vi "AutoCrossSubVi.vi"(0 "AutoDriveSpeed":dbl, 1 "DistanceAutoLineToBar":dbl, 2 "BarToShootLine":dbl, 3 "DriveDistanceDeadband":dbl, 5 "DriveDistanceVDeadband":dbl, 7 "VDeadband":dbl, 9 "EncoderDevRef 2":T1, 12 "Deadband":dbl, 13 "String":string, 14 "EncoderDevRef":T1) -> ()   [LabVIEW 2015]
uses:
  <vilib>/Rock Robotics/WPI/Encoder/WPI_EncoderDevRef.ctl
  <vilib>/Rock Robotics/SystemInterfaces/Encoder/FPGA_EncoderIdx.ctl
  <vilib>/Rock Robotics/SystemInterfaces/Counter/FPGA_CounterCtrSystemIndex.ctl
  <vilib>/Rock Robotics/WPI/Encoder/WPI_EncoderType.ctl
  AutoTask/Implementation/AutoTask Setpoints.ctl
  AutoTask/Implementation/AutoTask Operations.ctl
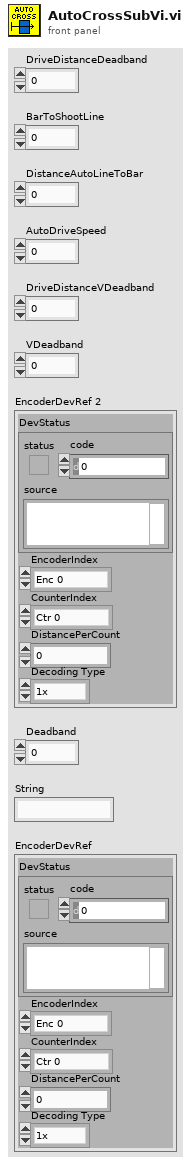
[diagram p1: front panel]
types:
  T1 = typedef "WPI_EncoderDevRef.ctl" = cluster{"DevStatus":errorcluster, "EncoderIndex":T2, "CounterIndex":T3, "DistancePerCount":dbl, "Decoding Type":T4}
  T2 = typedef "FPGA_EncoderIdx.ctl" = enum8{"Enc 0", "Enc 1", "Enc 2", "Enc 3", "Enc 4", "Enc 5", "Enc 6", "Enc 7", "Invalid"}
  T3 = typedef "FPGA_CounterCtrSystemIndex.ctl" = enum8{"Ctr 0", "Ctr 1", "Ctr 2", "Ctr 3", "Ctr 4", "Ctr 5", "Ctr 6", "Ctr 7", "Invalid"}
  T4 = typedef "WPI_EncoderType.ctl" = enum16{"1x", "2x", "4x"}
  T5 = typedef "AutoTask Setpoints.ctl" = cluster{"Operation":T6, "Setpoint":dbl, "Duration":dbl, "Speed":dbl, "Angle":dbl, "VDeadband":dbl, "Deadband":dbl}
  T6 = typedef "AutoTask Operations.ctl" = enum16{"Reserve", "Read Current", "Immediate", "DriveDistance", "AutoShoot", "FaceForward", "AutoAlign", "AutoTurn", "DriveToLine", "DriveToIncline", "DriveTillFlat"}
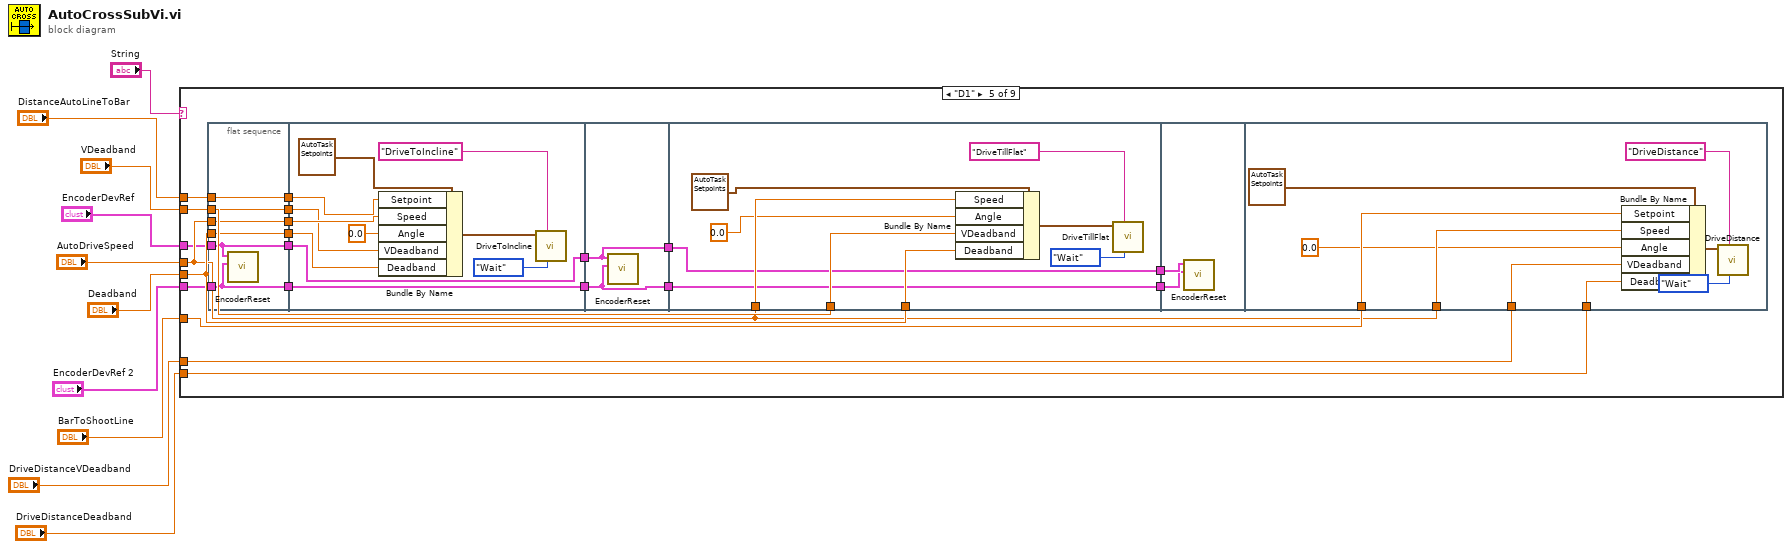
[diagram p0: block diagram]
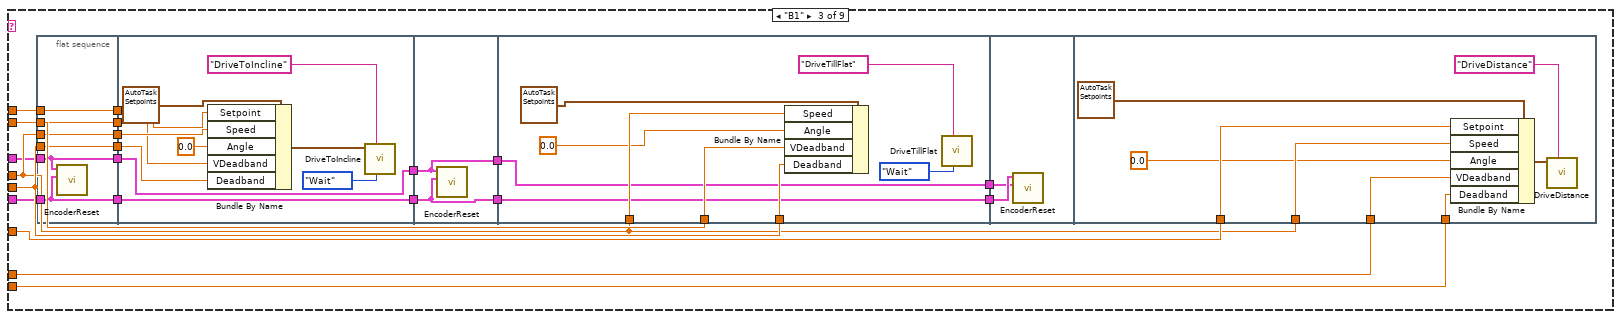
[diagram p4: hidden frame]
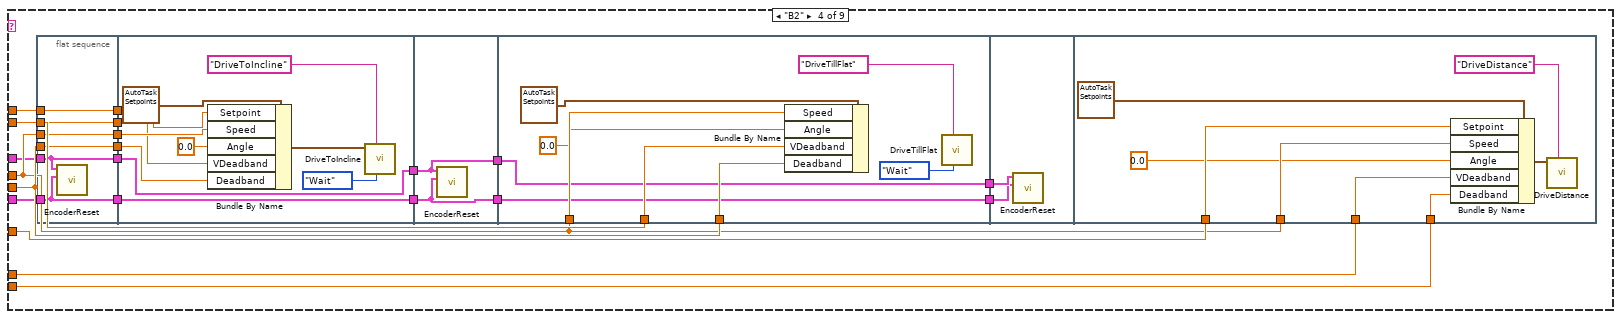
[diagram p5: hidden frame]
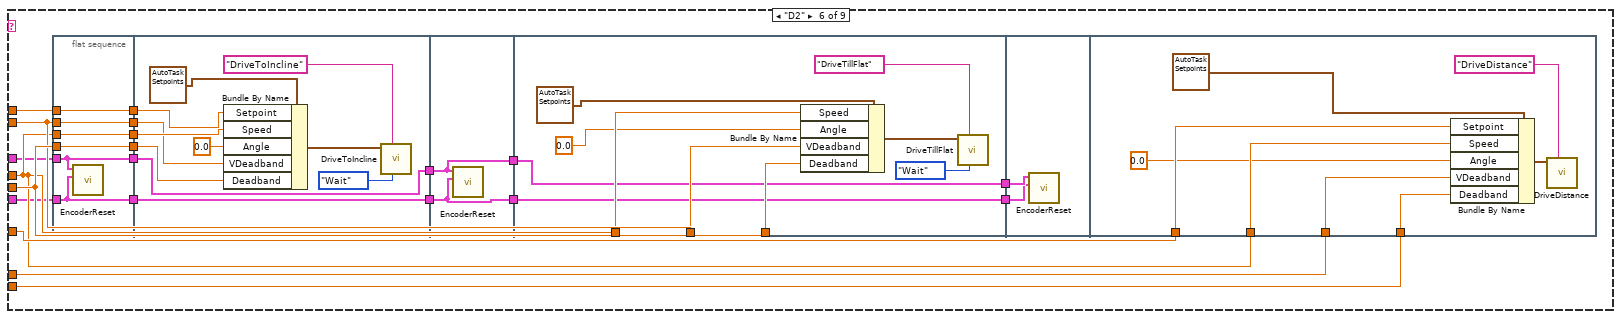
[diagram p6: hidden frame]
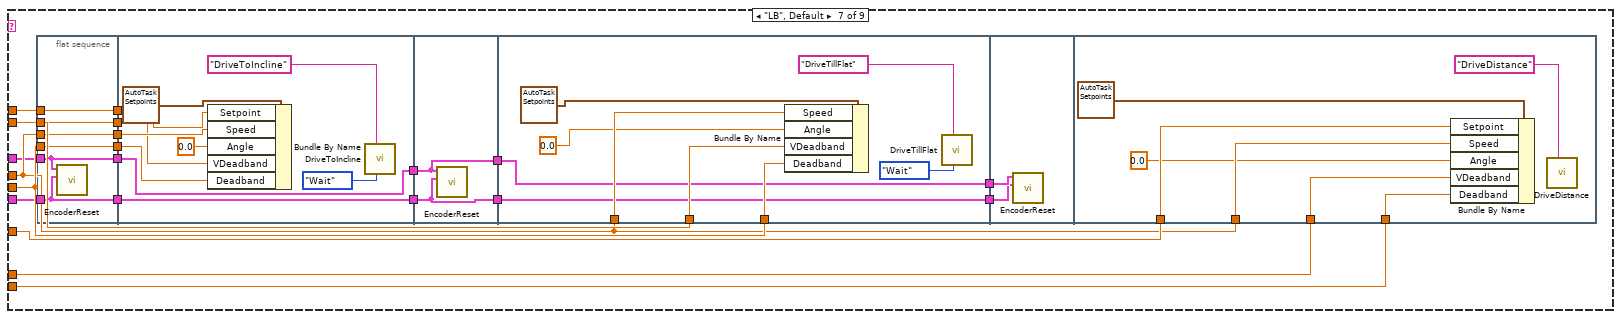
[diagram p7: hidden frame]
diagram:
  n1 = case shown="\"D1\"" "String" {
    tunnel: "DistanceAutoLineToBar" -> [_ _ w31 w90 w149 w210 w270 _ _]
    tunnel: "AutoDriveSpeed" -> [_ _ w27 w86 w145 w206 w266 _ _]
    tunnel: "VDeadband" -> [_ _ w29 w88 w147 w208 w268 _ _]
    tunnel: "Deadband" -> [_ _ w30 w89 w148 w209 w269 _ _]
    tunnel: "BarToShootLine" -> [_ _ w28 w87 w146 w207 w267 _ _]
    tunnel: "DriveDistanceDeadband" -> [_ _ w26 w85 w144 w205 w265 _ _]
    tunnel: "DriveDistanceVDeadband" -> [_ _ w25 w84 w143 w204 w264 _ _]
    tunnel: "EncoderDevRef 2" -> [_ _ w19 w78 w138 w198 w258 _ _]
    tunnel: "EncoderDevRef" -> [_ _ w20 w79 w137 w199 w259 _ _]
    frame "A1" {
    }
    frame "A2" {
    }
    frame "B1" {
      n2 = flat-sequence {
        tunnel: w30 -> [w34]
        tunnel: w29 -> [w35]
        tunnel: w27 -> [w36]
        tunnel: w31 -> [w37]
        tunnel: [w37] -> w24
        tunnel: [w36] -> w23
        tunnel: [w35] -> w22
        tunnel: [w34] -> w21
        tunnel: w20 -> [w33]
        tunnel: w19 -> [w32]
        tunnel: [w33] -> w18
        tunnel: [w32] -> w16
        tunnel: w24 -> [w45]
        tunnel: w23 -> [w44]
        tunnel: w22 -> [w42]
        tunnel: w21 -> [w41]
        tunnel: w18 -> [w39]
        tunnel: [w39] -> w17
        tunnel: w16 -> [w38]
        tunnel: [w38] -> w15
        tunnel: w17 -> [w49]
        tunnel: w15 -> [w50]
        tunnel: [w50] -> w14
        tunnel: [w49] -> w12
        tunnel: w27 -> [w56]
        tunnel: w30 -> [w54]
        tunnel: w29 -> [w53]
        tunnel: w14 -> [w52]
        tunnel: [w52] -> w13
        tunnel: w12 -> [w51]
        tunnel: [w51] -> w11
        tunnel: w13 -> [w61]
        tunnel: w11 -> [w60]
        tunnel: w28 -> [w66]
        tunnel: w27 -> [w65]
        tunnel: w26 -> [w63]
        tunnel: w25 -> [w62]
        frame #0 {
          n3 = call "EncoderReset.vi"("EncoderDevRef 2"=w32, "EncoderDevRef"=w33) -> ()  [unwired: 10 in]
        }
        frame #1 {
          n4 = Bundle By Name(cluster=T5 {"Operation"=enum."DriveToIncline", "Setpoint"=0.0, "Duration"=0.0, "Speed"=0.0, "Angle"=0.0, "VDeadband"=0.0, "Deadband"=0.0} ("SubSystem Data"), "Setpoint"=w45, "Speed"=w44, "Angle"=0.0, "VDeadband"=w42, "Deadband"=w41) -> (w47:T5)
          n5 = call "DriveToIncline.vi"("Synchronization"=enum16{"Start", "Wait"}."Wait", "Description"="DriveToIncline", "SubSystem Data"=w47) -> ()  [unwired: 8 in, 1 out]
        }
        frame #2 {
          n6 = call "EncoderReset.vi"("EncoderDevRef 2"=w50, "EncoderDevRef"=w49) -> ()  [unwired: 10 in]
        }
        frame #3 {
          n7 = Bundle By Name(cluster=T5 {"Operation"=enum."Reserve", "Setpoint"=0.0, "Duration"=0.0, "Speed"=0.0, "Angle"=0.0, "VDeadband"=0.0, "Deadband"=0.0} ("SubSystem Data"), "Speed"=w56, "Angle"=0.0, "VDeadband"=w53, "Deadband"=w54) -> ()  [unwired: 1 out]
          n8 = call "DriveTillFlat.vi"("Synchronization"=enum16{"Start", "Wait"}."Wait", "Description"="DriveTillFlat") -> ()  [unwired: 9 in, 1 out]
        }
        frame #4 {
          n9 = call "EncoderReset.vi"("EncoderDevRef 2"=w60, "EncoderDevRef"=w61) -> ()  [unwired: 10 in]
        }
        frame #5 {
          n10 = Bundle By Name(cluster=T5 {"Operation"=enum."DriveDistance", "Setpoint"=0.0, "Duration"=0.0, "Speed"=0.0, "Angle"=0.0, "VDeadband"=0.0, "Deadband"=0.0} ("SubSystem Data"), "Setpoint"=w66, "Speed"=w65, "Angle"=0.0, "VDeadband"=w62, "Deadband"=w63) -> (w68:T5)
          n11 = call "DriveDistance.vi"("Description"="DriveDistance", "SubSystem Data"=w68) -> ()  [unwired: 9 in, 1 out]
        }
      }
    }
    frame "B2" {
      n12 = flat-sequence {
        tunnel: w89 -> [w93]
        tunnel: w88 -> [w94]
        tunnel: w86 -> [w95]
        tunnel: w90 -> [w96]
        tunnel: [w96] -> w83
        tunnel: [w95] -> w82
        tunnel: [w94] -> w81
        tunnel: [w93] -> w80
        tunnel: w79 -> [w92]
        tunnel: w78 -> [w91]
        tunnel: [w92] -> w77
        tunnel: [w91] -> w75
        tunnel: w83 -> [w104]
        tunnel: w82 -> [w103]
        tunnel: w81 -> [w101]
        tunnel: w80 -> [w100]
        tunnel: w77 -> [w98]
        tunnel: [w98] -> w76
        tunnel: w75 -> [w97]
        tunnel: [w97] -> w74
        tunnel: w76 -> [w109]
        tunnel: w74 -> [w108]
        tunnel: [w109] -> w73
        tunnel: [w108] -> w71
        tunnel: w86 -> [w115]
        tunnel: w89 -> [w113]
        tunnel: w88 -> [w112]
        tunnel: w73 -> [w111]
        tunnel: [w111] -> w72
        tunnel: w71 -> [w110]
        tunnel: [w110] -> w70
        tunnel: w72 -> [w120]
        tunnel: w70 -> [w119]
        tunnel: w87 -> [w125]
        tunnel: w86 -> [w124]
        tunnel: w85 -> [w122]
        tunnel: w84 -> [w121]
        frame #0 {
          n13 = call "EncoderReset.vi"("EncoderDevRef 2"=w91, "EncoderDevRef"=w92) -> ()  [unwired: 10 in]
        }
        frame #1 {
          n14 = Bundle By Name(cluster=T5 {"Operation"=enum."DriveToIncline", "Setpoint"=0.0, "Duration"=0.0, "Speed"=0.0, "Angle"=0.0, "VDeadband"=0.0, "Deadband"=0.0} ("SubSystem Data"), "Setpoint"=w104, "Speed"=w103, "Angle"=0.0, "VDeadband"=w101, "Deadband"=w100) -> (w106:T5)
          n15 = call "DriveToIncline.vi"("Synchronization"=enum16{"Start", "Wait"}."Wait", "Description"="DriveToIncline", "SubSystem Data"=w106) -> ()  [unwired: 8 in, 1 out]
        }
        frame #2 {
          n16 = call "EncoderReset.vi"("EncoderDevRef 2"=w108, "EncoderDevRef"=w109) -> ()  [unwired: 10 in]
        }
        frame #3 {
          n17 = Bundle By Name(cluster=T5 {"Operation"=enum."Reserve", "Setpoint"=0.0, "Duration"=0.0, "Speed"=0.0, "Angle"=0.0, "VDeadband"=0.0, "Deadband"=0.0} ("SubSystem Data"), "Speed"=w115, "Angle"=0.0, "VDeadband"=w112, "Deadband"=w113) -> ()  [unwired: 1 out]
          n18 = call "DriveTillFlat.vi"("Synchronization"=enum16{"Start", "Wait"}."Wait", "Description"="DriveTillFlat") -> ()  [unwired: 9 in, 1 out]
        }
        frame #4 {
          n19 = call "EncoderReset.vi"("EncoderDevRef 2"=w119, "EncoderDevRef"=w120) -> ()  [unwired: 10 in]
        }
        frame #5 {
          n20 = Bundle By Name(cluster=T5 {"Operation"=enum."DriveDistance", "Setpoint"=0.0, "Duration"=0.0, "Speed"=0.0, "Angle"=0.0, "VDeadband"=0.0, "Deadband"=0.0} ("SubSystem Data"), "Setpoint"=w125, "Speed"=w124, "Angle"=0.0, "VDeadband"=w121, "Deadband"=w122) -> (w127:T5)
          n21 = call "DriveDistance.vi"("Description"="DriveDistance", "SubSystem Data"=w127) -> ()  [unwired: 9 in, 1 out]
        }
      }
    }
    frame "D1" {
      n22 = flat-sequence {
        tunnel: w148 -> [w152]
        tunnel: w147 -> [w153]
        tunnel: w145 -> [w154]
        tunnel: w149 -> [w155]
        tunnel: [w155] -> w142
        tunnel: [w154] -> w141
        tunnel: [w153] -> w140
        tunnel: [w152] -> w139
        tunnel: w138 -> [w150]
        tunnel: w137 -> [w151]
        tunnel: [w151] -> w136
        tunnel: [w150] -> w135
        tunnel: w142 -> [w163]
        tunnel: w141 -> [w162]
        tunnel: w140 -> [w160]
        tunnel: w139 -> [w159]
        tunnel: w136 -> [w157]
        tunnel: w135 -> [w156]
        tunnel: [w157] -> w134
        tunnel: [w156] -> w133
        tunnel: w134 -> [w168]
        tunnel: w133 -> [w167]
        tunnel: [w168] -> w132
        tunnel: [w167] -> w130
        tunnel: w145 -> [w175]
        tunnel: w148 -> [w173]
        tunnel: w147 -> [w172]
        tunnel: w132 -> [w171]
        tunnel: [w171] -> w131
        tunnel: w130 -> [w170]
        tunnel: [w170] -> w129
        tunnel: w131 -> [w180]
        tunnel: w129 -> [w179]
        tunnel: w146 -> [w187]
        tunnel: w145 -> [w186]
        tunnel: w144 -> [w184]
        tunnel: w143 -> [w183]
        frame #0 {
          n23 = call "EncoderReset.vi"("EncoderDevRef 2"=w150, "EncoderDevRef"=w151) -> ()  [unwired: 10 in]
        }
        frame #1 {
          n24 = Bundle By Name(cluster=T5 {"Operation"=enum."DriveToIncline", "Setpoint"=0.0, "Duration"=0.0, "Speed"=0.0, "Angle"=0.0, "VDeadband"=0.0, "Deadband"=0.0} ("SubSystem Data"), "Setpoint"=w163, "Speed"=w162, "Angle"=0.0, "VDeadband"=w160, "Deadband"=w159) -> (w165:T5)
          n25 = call "DriveToIncline.vi"("Synchronization"=enum16{"Start", "Wait"}."Wait", "Description"="DriveToIncline", "SubSystem Data"=w165) -> ()  [unwired: 8 in, 1 out]
        }
        frame #2 {
          n26 = call "EncoderReset.vi"("EncoderDevRef 2"=w167, "EncoderDevRef"=w168) -> ()  [unwired: 10 in]
        }
        frame #3 {
          n27 = Bundle By Name(cluster=T5 {"Operation"=enum."Reserve", "Setpoint"=0.0, "Duration"=0.0, "Speed"=0.0, "Angle"=0.0, "VDeadband"=0.0, "Deadband"=0.0} ("SubSystem Data"), "Speed"=w175, "Angle"=0.0, "VDeadband"=w172, "Deadband"=w173) -> (w169:T5)
          n28 = call "DriveTillFlat.vi"("Synchronization"=enum16{"Start", "Wait"}."Wait", "Description"="DriveTillFlat", "SubSystem Data"=w169) -> ()  [unwired: 8 in, 1 out]
        }
        frame #4 {
          n29 = call "EncoderReset.vi"("EncoderDevRef 2"=w179, "EncoderDevRef"=w180) -> ()  [unwired: 10 in]
        }
        frame #5 {
          n30 = Bundle By Name(cluster=T5 {"Operation"=enum."DriveDistance", "Setpoint"=0.0, "Duration"=0.0, "Speed"=0.0, "Angle"=0.0, "VDeadband"=0.0, "Deadband"=0.0} ("SubSystem Data"), "Setpoint"=w187, "Speed"=w186, "Angle"=0.0, "VDeadband"=w183, "Deadband"=w184) -> (w182:T5)
          n31 = call "DriveDistance.vi"("Synchronization"=enum16{"Start", "Wait"}."Wait", "Description"="DriveDistance", "SubSystem Data"=w182) -> ()  [unwired: 8 in, 1 out]
        }
      }
    }
    frame "D2" {
      n32 = flat-sequence {
        tunnel: w209 -> [w213]
        tunnel: w208 -> [w214]
        tunnel: w206 -> [w215]
        tunnel: w210 -> [w216]
        tunnel: [w216] -> w203
        tunnel: [w215] -> w202
        tunnel: [w214] -> w201
        tunnel: [w213] -> w200
        tunnel: w199 -> [w212]
        tunnel: w198 -> [w211]
        tunnel: [w212] -> w197
        tunnel: [w211] -> w195
        tunnel: w203 -> [w226]
        tunnel: w202 -> [w225]
        tunnel: w201 -> [w223]
        tunnel: w200 -> [w222]
        tunnel: w197 -> [w220]
        tunnel: [w220] -> w196
        tunnel: w195 -> [w219]
        tunnel: [w219] -> w194
        tunnel: w196 -> [w229]
        tunnel: w194 -> [w228]
        tunnel: [w229] -> w193
        tunnel: [w228] -> w191
        tunnel: w206 -> [w236]
        tunnel: w209 -> [w234]
        tunnel: w208 -> [w233]
        tunnel: w193 -> [w232]
        tunnel: [w232] -> w192
        tunnel: w191 -> [w231]
        tunnel: [w231] -> w190
        tunnel: w192 -> [w241]
        tunnel: w190 -> [w240]
        tunnel: w207 -> [w248]
        tunnel: w206 -> [w247]
        tunnel: w205 -> [w245]
        tunnel: w204 -> [w244]
        frame #0 {
          n33 = call "EncoderReset.vi"("EncoderDevRef 2"=w211, "EncoderDevRef"=w212) -> ()  [unwired: 10 in]
        }
        frame #1 {
          n34 = Bundle By Name(cluster=T5 {"Operation"=enum."Reserve", "Setpoint"=0.0, "Duration"=0.0, "Speed"=0.0, "Angle"=0.0, "VDeadband"=0.0, "Deadband"=0.0} ("SubSystem Data"), "Setpoint"=w226, "Speed"=w225, "Angle"=0.0, "VDeadband"=w223, "Deadband"=w222) -> (w217:T5)
          n35 = call "DriveToIncline.vi"("Synchronization"=enum16{"Start", "Wait"}."Wait", "Description"="DriveToIncline", "SubSystem Data"=w217) -> ()  [unwired: 8 in, 1 out]
        }
        frame #2 {
          n36 = call "EncoderReset.vi"("EncoderDevRef 2"=w228, "EncoderDevRef"=w229) -> ()  [unwired: 10 in]
        }
        frame #3 {
          n37 = Bundle By Name(cluster=T5 {"Operation"=enum."Reserve", "Setpoint"=0.0, "Duration"=0.0, "Speed"=0.0, "Angle"=0.0, "VDeadband"=0.0, "Deadband"=0.0} ("SubSystem Data"), "Speed"=w236, "Angle"=0.0, "VDeadband"=w233, "Deadband"=w234) -> (w230:T5)
          n38 = call "DriveTillFlat.vi"("Synchronization"=enum16{"Start", "Wait"}."Wait", "Description"="DriveTillFlat", "SubSystem Data"=w230) -> ()  [unwired: 8 in, 1 out]
        }
        frame #4 {
          n39 = call "EncoderReset.vi"("EncoderDevRef 2"=w240, "EncoderDevRef"=w241) -> ()  [unwired: 10 in]
        }
        frame #5 {
          n40 = Bundle By Name(cluster=T5 {"Operation"=enum."Reserve", "Setpoint"=0.0, "Duration"=0.0, "Speed"=0.0, "Angle"=0.0, "VDeadband"=0.0, "Deadband"=0.0} ("SubSystem Data"), "Setpoint"=w248, "Speed"=w247, "Angle"=0.0, "VDeadband"=w244, "Deadband"=w245) -> (w242:T5)
          n41 = call "DriveDistance.vi"("Description"="DriveDistance", "SubSystem Data"=w242) -> ()  [unwired: 9 in, 1 out]
        }
      }
    }
    frame "LB", Default {
      n42 = flat-sequence {
        tunnel: w269 -> [w273]
        tunnel: w268 -> [w274]
        tunnel: w266 -> [w275]
        tunnel: w270 -> [w276]
        tunnel: [w276] -> w263
        tunnel: [w275] -> w262
        tunnel: [w274] -> w261
        tunnel: [w273] -> w260
        tunnel: w259 -> [w272]
        tunnel: w258 -> [w271]
        tunnel: [w272] -> w257
        tunnel: [w271] -> w255
        tunnel: w263 -> [w284]
        tunnel: w262 -> [w283]
        tunnel: w261 -> [w281]
        tunnel: w260 -> [w280]
        tunnel: w257 -> [w278]
        tunnel: [w278] -> w256
        tunnel: w255 -> [w277]
        tunnel: [w277] -> w254
        tunnel: w256 -> [w288]
        tunnel: w254 -> [w287]
        tunnel: [w288] -> w253
        tunnel: [w287] -> w251
        tunnel: w266 -> [w294]
        tunnel: w269 -> [w292]
        tunnel: w268 -> [w291]
        tunnel: w253 -> [w290]
        tunnel: [w290] -> w252
        tunnel: w251 -> [w289]
        tunnel: [w289] -> w250
        tunnel: w252 -> [w299]
        tunnel: w250 -> [w298]
        tunnel: w267 -> [w304]
        tunnel: w266 -> [w303]
        tunnel: w265 -> [w301]
        tunnel: w264 -> [w300]
        frame #0 {
          n43 = call "EncoderReset.vi"("EncoderDevRef 2"=w271, "EncoderDevRef"=w272) -> ()  [unwired: 10 in]
        }
        frame #1 {
          n44 = Bundle By Name(cluster=T5 {"Operation"=enum."DriveToIncline", "Setpoint"=0.0, "Duration"=0.0, "Speed"=0.0, "Angle"=0.0, "VDeadband"=0.0, "Deadband"=0.0} ("SubSystem Data"), "Setpoint"=w284, "Speed"=w283, "Angle"=0.0, "VDeadband"=w281, "Deadband"=w280) -> ()  [unwired: 1 out]
          n45 = call "DriveToIncline.vi"("Synchronization"=enum16{"Start", "Wait"}."Wait", "Description"="DriveToIncline") -> ()  [unwired: 9 in, 1 out]
        }
        frame #2 {
          n46 = call "EncoderReset.vi"("EncoderDevRef 2"=w287, "EncoderDevRef"=w288) -> ()  [unwired: 10 in]
        }
        frame #3 {
          n47 = Bundle By Name(cluster=T5 {"Operation"=enum."Reserve", "Setpoint"=0.0, "Duration"=0.0, "Speed"=0.0, "Angle"=0.0, "VDeadband"=0.0, "Deadband"=0.0} ("SubSystem Data"), "Speed"=w294, "Angle"=0.0, "VDeadband"=w291, "Deadband"=w292) -> ()  [unwired: 1 out]
          n48 = call "DriveTillFlat.vi"("Synchronization"=enum16{"Start", "Wait"}."Wait", "Description"="DriveTillFlat") -> ()  [unwired: 9 in, 1 out]
        }
        frame #4 {
          n49 = call "EncoderReset.vi"("EncoderDevRef 2"=w298, "EncoderDevRef"=w299) -> ()  [unwired: 10 in]
        }
        frame #5 {
          n50 = Bundle By Name(cluster=T5 {"Operation"=enum."DriveDistance", "Setpoint"=0.0, "Duration"=0.0, "Speed"=0.0, "Angle"=0.0, "VDeadband"=0.0, "Deadband"=0.0} ("SubSystem Data"), "Setpoint"=w304, "Speed"=w303, "Angle"=0.0, "VDeadband"=w300, "Deadband"=w301) -> ()  [unwired: 1 out]
          n51 = call "DriveDistance.vi"("Description"="DriveDistance") -> ()  [unwired: 10 in, 1 out]
        }
      }
    }
    frame "C1" {
    }
    frame "C2" {
    }
  }
